vi "公式计算.vi"() -> ()   [LabVIEW 2022 SP3]
uses:
  <vilib>/express/express arith-compare/Formula/XNode/ExpressFormulaBlockNode.xnode
panel:
  in  "公式":string
  in  "停止":bool
  out "结果":dbl
  in  "输入":dbl
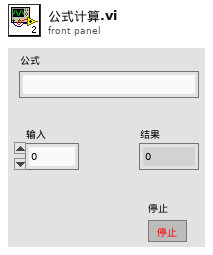
[diagram p1: front panel]
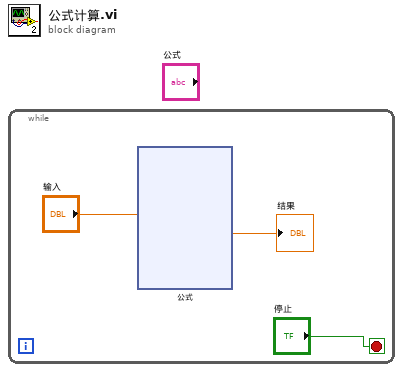
[diagram p0: block diagram]
diagram:
  n1 = while {
    stop <- "停止" stop-if-true
    n2 = xnode "公式"("X1"="输入") -> ("结果"=→"结果":dbl)  [unwired: 1 in, 1 out]
  }
